vi "BinF_ReadHeader.vi"(8 "error in":errorcluster, 11 "refnum":refnum<file>) -> (0 "error out":errorcluster, 3 "refnum out":refnum<file>, 5 "BinF File Settings":T1={"Version"=2, "Data Representation"=enum."I16", "# columns (samples per channel)"=300, "# rows (channels)"=150, "# pre-trigger samples"=20, "Sample rate"=1000.0, "ADC offset"=256.0, "Scale factor"=0.001})   [LabVIEW 2021]
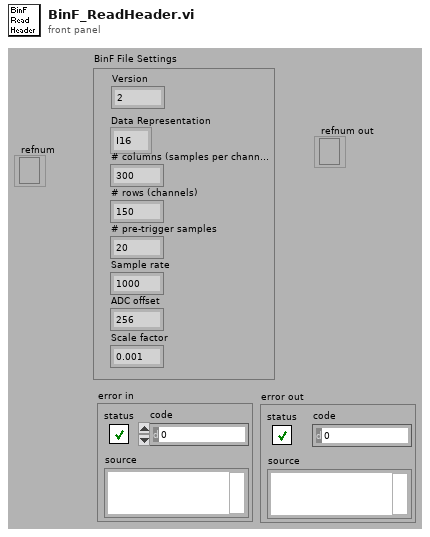
[diagram p1: front panel]
types:
  T1 = cluster{"Version":i16, "Data Representation":enum16{"Undefined", "I8", "I16", "I32", "I64", "U8", "U16", "U32", "U64", "SGL", "DBL", "EXT"}, "# columns (samples per channel)":i64, "# rows (channels)":i64, "# pre-trigger samples":i64, "Sample rate":dbl, "ADC offset":dbl, "Scale factor":dbl}
  T2 = enum16{"Undefined", "I8", "I16", "I32", "I64", "U8", "U16", "U32", "U64", "SGL", "DBL", "EXT"}
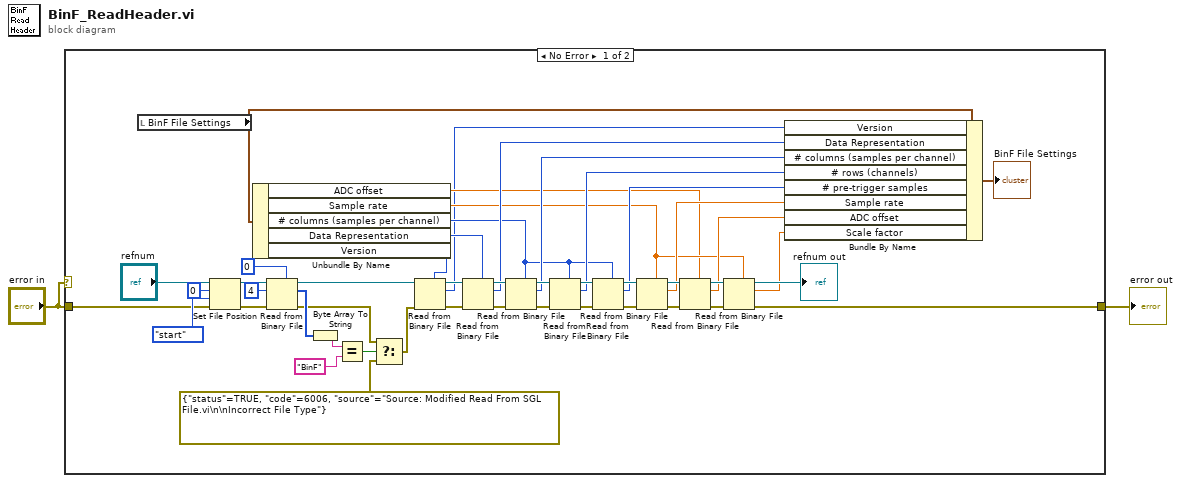
[diagram p0: block diagram]
diagram:
  n1 = case shown="No Error" "error in" {
    tunnel: "error in" -> [w36 w50]
    tunnel: [w33 w50] -> w2
    frame No Error {
      n2 = local read "BinF File Settings"() -> (w12:T1)
      n3 = Set File Position(offset (in bytes) (0)=i64 0, refnum="refnum", from (0:start)=enum16{"start", "end", "current"}."start", error in=w36) -> (refnum out=w30:refnum<file>, error out=w31:errorcluster)
      n4 = Unbundle By Name(w12) -> ("ADC offset"=w8:dbl, "Sample rate"=w9:dbl, "# columns (samples per channel)"=w10:i64, "Data Representation"=w11:T2, "Version"=w6:i16)
      n5 = Read from Binary File(5:u8 0, 8:w31, 10:4 ("count"), 11:w30) -> (0:w22:errorcluster, 2:w27:u8[], 3:w5:refnum<file>)  [unwired: 3 out]
      n6 = Byte Array To String(unsigned byte array=w27) -> (string=w26:string)
      n7 = Equal?(x=w26, y="BinF") -> (x = y?=w24:bool)
      n8 = Select(t=w22, s=w24, f=errorcluster {"status"=TRUE, "code"=6006, "source"="Source: Modified Read From SGL File.vi\n\nIncorrect File Type"} ("error out")) -> (s? t:f=w21:errorcluster)
      n9 = Read from Binary File(5:w6, 8:w21, 11:w5) -> (0:w7:errorcluster, 2:w3:i16, 3:w4:refnum<file>)  [unwired: 4 out]
      n10 = Read from Binary File(5:w11, 8:w7, 11:w4) -> (0:w48:errorcluster, 2:w20:T2, 3:w49:refnum<file>)  [unwired: 4 out]
      n11 = Read from Binary File(5:w10, 8:w48, 11:w49) -> (0:w47:errorcluster, 2:w18:i64, 3:w46:refnum<file>)  [unwired: 4 out]
      n12 = Read from Binary File(5:w10, 8:w47, 11:w46) -> (0:w45:errorcluster, 2:w17:i64, 3:w44:refnum<file>)  [unwired: 4 out]
      n13 = Read from Binary File(5:w10, 8:w45, 11:w44) -> (0:w43:errorcluster, 2:w16:i64, 3:w42:refnum<file>)  [unwired: 4 out]
      n14 = Read from Binary File(5:w9, 8:w43, 11:w42) -> (0:w41:errorcluster, 2:w15:dbl, 3:w40:refnum<file>)  [unwired: 4 out]
      n15 = Read from Binary File(5:w8, 8:w41, 11:w40) -> (0:w35:errorcluster, 2:w14:dbl, 3:w34:refnum<file>)  [unwired: 4 out]
      n16 = Read from Binary File(5:w9, 8:w35, 11:w34) -> (0:w33:errorcluster, 2:w13:dbl, 3:→"refnum out":refnum<file>)  [unwired: 4 out]
      n17 = Bundle By Name(cluster=w12, "Version"=w3, "Data Representation"=w20, "# columns (samples per channel)"=w18, "# rows (channels)"=w17, "# pre-trigger samples"=w16, "Sample rate"=w15, "ADC offset"=w14, "Scale factor"=w13) -> (→"BinF File Settings":T1)
    }
    frame Error {
    }
  }
  "error out" <- w2
